vi "UpdateValues.vi"(8 "error in (no error)":errorcluster, 9 "history values":T2[](array[typedef]), 10 "buffer size":i32, 11 "map":T1) -> (0 "error out":errorcluster, 1 "history values out":T2[](array[typedef]))   [LabVIEW 2017, in "TestPanel.lvlib"]
uses:
  <vilib>/addons/InsightCM/Devices/Shared/Common/TestPanel/TestPanel.lvlib
  <vilib>/addons/InsightCM/MessageBus/Base/controls/TestPanelTimeSeries.ctl
  <vilib>/addons/InsightCM/MessageBus/Base/controls/TestPanelValue.ctl
  <vilib>/addons/PointValueMap/controls/PointMap.ctl
  <vilib>/addons/PointValueMap/subVIs/Point_Read_double.vi
  <vilib>/addons/PointValueMap/PointValueMap.lvlib
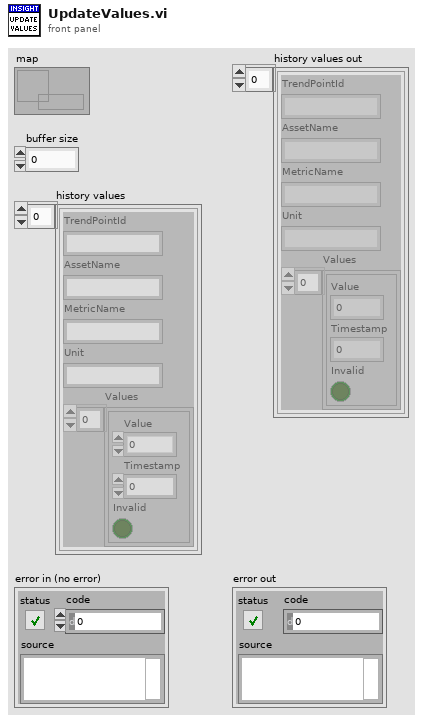
[diagram p1: front panel]
types:
  T1 = typedef "PointValueMap.lvlib/PointMap.ctl" = refnum<data-value>
  T2 = typedef "TestPanelTimeSeries.ctl" = cluster{"TrendPointId":string, "AssetName":string, "MetricName":string, "Unit":string, "Values":T3[]}
  T3 = typedef "TestPanelValue.ctl" = cluster{"Value":dbl, "Timestamp":i64, "Invalid":bool}
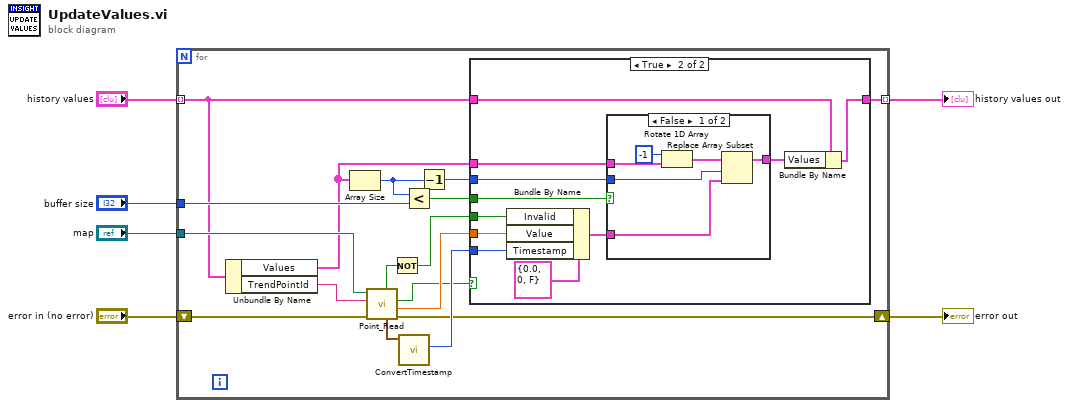
[diagram p0: block diagram]
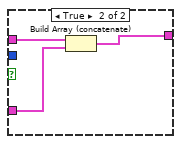
[diagram p3: hidden frame]
diagram:
  n1 = for {
    tunnel: "history values" -> [w11] mode=indexing
    shift-right: [w8] -> w2
    shift-left: "error in (no error)" -> [w23]
    tunnel: "map" -> [w21]
    tunnel: "buffer size" -> [w15]
    tunnel: [w10] -> w3 mode=indexing
    n2 = Unbundle By Name(w11) -> ("Values"=w9:T3[], "TrendPointId"=w22:string)
    n3 = Array Size(array=w9) -> (size(s)=w13:i32)
    n4 = call-poly <vilib>:"Point_Read.vi"("Error In"=w23, "Tag"=w22, "Map"=w21) -> ("Error Out"=w8:errorcluster, "Value"=w18:dbl, "Found?"=w7:bool, "Time Stamp"=w17:timestamp, "Valid?"=w20:bool)  [unwired: 3 in, 1 out]
    n5 = Not(x=w20) -> (.not. x?=w19:bool)
    n6 = call <vilib>:"ConvertTimestamp.vi"("Time Stamp"=w17) -> ("Timestamp out"=w16:i64)  [unwired: 10 in]
    n7 = Less?(x=w13, y=w15) -> (x < y?=w14:bool)
    n8 = Decrement(x=w13) -> (x-1=w12:i32)
    n9 = case shown="True" w7 {
      tunnel: w19 -> [_ w34]
      tunnel: w18 -> [_ w33]
      tunnel: w16 -> [_ w32]
      tunnel: w14 -> [_ w30]
      tunnel: w12 -> [_ w29]
      tunnel: w11 -> [w24 w28]
      tunnel: [w24 w26] -> w10
      tunnel: w9 -> [_ w25]
      frame False {
      }
      frame True {
        n10 = Bundle By Name(cluster=T3 {"Value"=0.0, "Timestamp"=0, "Invalid"=FALSE} ("Value"), "Invalid"=w34, "Value"=w33, "Timestamp"=w32) -> (w31:T3)
        n11 = case shown="False" w30 {
          tunnel: w31 -> [w38 w44]
          tunnel: w25 -> [w41 w43]
          tunnel: w29 -> [w37 _]
          tunnel: [w36 w42] -> w27
          frame False {
            n12 = Rotate 1D Array(1:w41, 2:-1 ("n")) -> (0:w39:T3[])
            n13 = Replace Array Subset(array=w39, new element=w38, index=w37) -> (w36:T3[])
          }
          frame True {
            n14 = Build Array (concatenate)(w43, w44) -> (w42:T3[])
          }
        }
        n15 = Bundle By Name(cluster=w28, "Values"=w27) -> (w26:T2)
      }
    }
  }
  "history values out" <- w3
  "error out" <- w2
